vi "Read Measurement Data (Raw 1Chan).vi"(0 "VISA resource name":refnum<visa-resource-name>, 5 "Channel (1)":string="0001", 11 "error in (no error)":errorcluster) -> (2 "Date Time":timestamp=timestamp(3345116400 s since 1904-01-01) format="%<%H:%M:%S%3u\n%x>T", 4 "VISA resource name out":refnum<visa-resource-name>, 6 "Channel":string, 8 "Data":i32, 10 "Data Status":i32(ring) items=["Normal", "Differential Input", "Skip", "Over", "Error", "Burnout", "Power Failure"], 13 "Alarm Status":i32[](array[ring]) items=["No Alarm", "High Limit Alarm (H)", "Low Limit Alarm (L)", "Difference High Limit Alarm (h)", "Difference Low Limit Alarm (l)", "High Limit on Rate-of-change Alarm (R)", "Low Limit on Rate-of-change Alarm (r)", "Delay High Limit Alarm (T)", "Delay Low Limit Alarm (t)"], 14 "Data Type":i32(ring) items=["", "INT", "FLOAT"], 15 "error out":errorcluster)   [LabVIEW 2020, in "Yokogawa GX Series.lvlib"]
doc: "This VI reads the raw measurement data by Binary."
uses:
  <instrlib>/Yokogawa GX Series/Yokogawa GX Series.lvlib
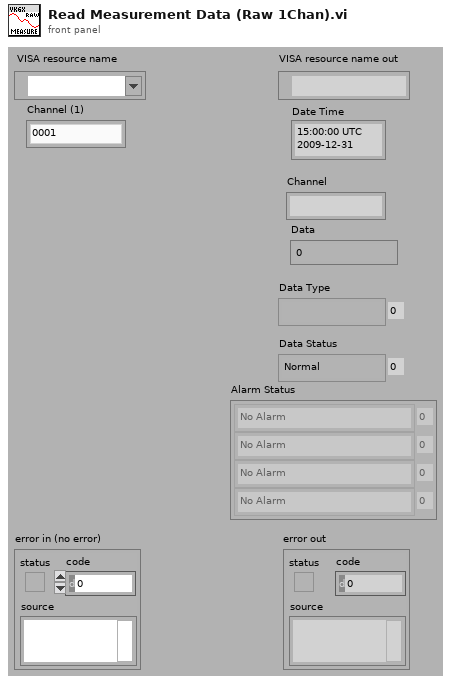
[diagram p1: front panel]
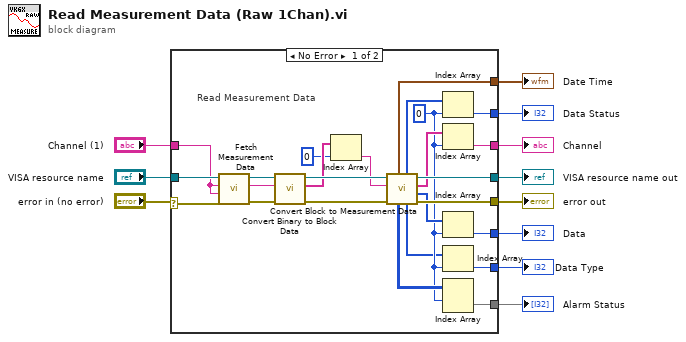
[diagram p0: block diagram]
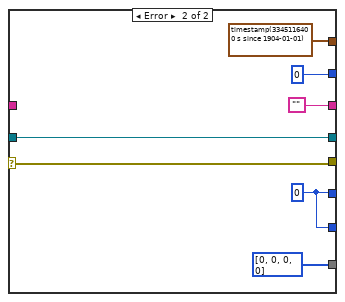
[diagram p2: hidden frame]
diagram:
  n1 = case shown="No Error" "error in (no error)" {
    selector: "error in (no error)" -> [w15 w42]
    tunnel: "VISA resource name" -> [w36 w43]
    tunnel: [w35 w43] -> w10
    tunnel: [w34 w42] -> w9
    tunnel: [w33 timestamp(3345116400 s since 1904-01-01)] -> w8
    tunnel: [w32 ""] -> w7
    tunnel: [w31 w37] -> w6
    tunnel: [w30 i32[] [0, 0, 0, 0]] -> w5
    tunnel: [w29 0] -> w4
    tunnel: "Channel (1)" -> [w28 _]
    tunnel: [w12 w37] -> w1
    frame No Error {
      w14 = 0
      # "Read Measurement Data"
      n2 = call <instrlib>:"Fetch Measurement Data.vi"("error in (no error)"=w15, "End Channel (1)"=w28, "Start Channel (1)"=w28, "VISA resource name"=w36) -> ("error out"=w23:errorcluster, "Measurement Data"=w25:string, "VISA resource name out"=w24:refnum<visa-resource-name>)  [unwired: 1 in, 4 out]
      n3 = call <instrlib>:"Convert Binary to Block Data.vi"("error in (no error)"=w23, "Measurement Binary Data (\"\")"=w25, "VISA resource name"=w24) -> ("error out"=w26:errorcluster, "Measurement Block Data"=w22:string[], "VISA resource name out"=w27:refnum<visa-resource-name>)  [unwired: 6 out]
      n4 = Index Array(array=w22, index=0) -> (element=w21:string)
      n5 = call <instrlib>:"Convert Block to Measurement Data.vi"("error in (no error)"=w26, "Measurement Block Data (\"\")"=w21, "VISA resource name"=w27) -> ("error out"=w34:errorcluster, "Data"=w18:i32[], "Channel"=w19:string[], "VISA resource name out"=w35:refnum<visa-resource-name>, "Data Type"=w13:i32[], "Data Status"=w16:i32[], "Alarm Status"=w17:i32[][], "Date Time"=w33:timestamp)  [unwired: 1 out]
      n6 = Index Array(array=w16, index=w14) -> (element=w29:i32)
      n7 = Index Array(array=w19, index=w14) -> (element=w32:string)
      n8 = Index Array(array=w18, index=w14) -> (element=w31:i32)
      n9 = Index Array(array=w13, index=w14) -> (element=w12:i32)
      n10 = Index Array(array=w17, index (row)=w14) -> (element=w30:i32[])  [unwired: 1 in]
    }
    frame Error {
      w37 = 0
    }
  }
  "error out" <- w9
  "VISA resource name out" <- w10
  "Channel" <- w7
  "Alarm Status" <- w5
  "Date Time" <- w8
  "Data" <- w6
  "Data Status" <- w4
  "Data Type" <- w1
